vi "dead lock.vi"   [LabVIEW 2010]
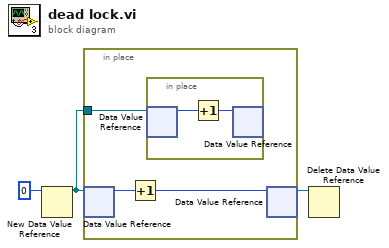
[diagram p0: block diagram]
diagram:
  n1 = New Data Value Reference(data value=0) -> (data value reference=w1:refnum<data-value>)  [unwired: 1 in, 1 out]
  n2 = in-place {
    in-place-border: w1 -> [w4]
    n3 = in-place-dvr #1(w1) -> (w6:i32)  [unwired: 1 out]
    n4 = Increment(x=w6) -> (x+1=w5:i32)
    n5 = in-place {
      n6 = in-place-dvr #2(w4) -> (w8:i32)  [unwired: 1 out]
      n7 = Increment(x=w8) -> (x+1=w7:i32)
      n8 = in-place-dvr #2(w7) -> ()  [unwired: 2 out]
    }
    n9 = in-place-dvr #1(w5) -> (w2:refnum<data-value>)  [unwired: 1 out]
  }
  n10 = Delete Data Value Reference(data value reference=w2) -> ()  [unwired: 1 in, 2 out]
